vi "InitConnection.vi"(8 "error in (no error)":errorcluster, 11 "TCS in":refnum<class "TCS.lvclass">) -> (0 "error out":errorcluster, 3 "TCS out":refnum<class "TCS.lvclass">)   [LabVIEW 2018, in "TCS.lvclass"]
uses:
  TCS.lvclass
  Server/Server.lvclass
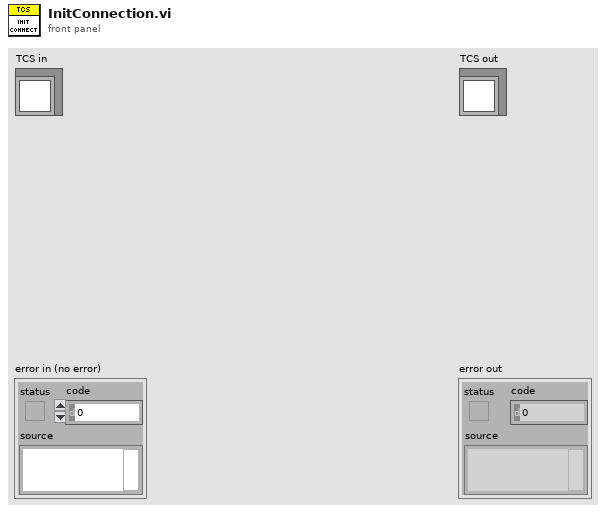
[diagram p1: front panel]
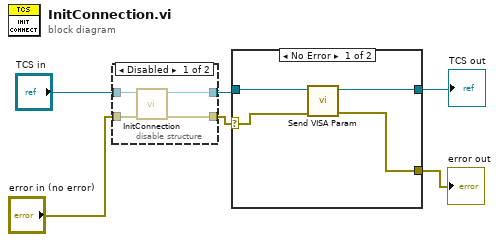
[diagram p0: block diagram]
diagram:
  n1 = disable-structure shown="Disabled" {
    disable-tunnel: [w10 w11] -> w3
    disable-tunnel: [w9 w12] -> w4
    disable-tunnel: "error in (no error)" -> [w8 w11]
    disable-tunnel: "TCS in" -> [w7 w12]
    frame Disabled {
      n2 = call-parent "InitConnection.vi"("error in (no error)"=w8, "Server in"=w7) -> ("error out"=w10:errorcluster, "Server out"=w9:refnum<class "TCS.lvclass">)  [unwired: 8 in]
    }
    frame Enabled {
    }
  }
  n3 = case shown="No Error" w3 {
    selector: w3 -> [w15 w17]
    tunnel: w4 -> [w16 w18]
    tunnel: [w14 w17] -> w1
    tunnel: [w13 w18] -> w2
    frame No Error {
      n4 = call-dynamic "Send VISA Param.vi"("error in (no error)"=w15, "Server in"=w16) -> ("error out"=w14:errorcluster, "Server out"=w13:refnum<class "TCS.lvclass">)  [unwired: 8 in]
    }
    frame Error {
    }
  }
  "error out" <- w1
  "TCS out" <- w2
